vi "pp2_StimListPartition5.vi"(0 "Session List (Hidden variable)":u8[](array[numeric])=[0, 1, 2, 3, 4, 5, 6, 7, 8, 9, 10, 11, 12, 13, 14, 15, 100]) -> (7 "Session list display":string[][](table))   [LabVIEW 2013]
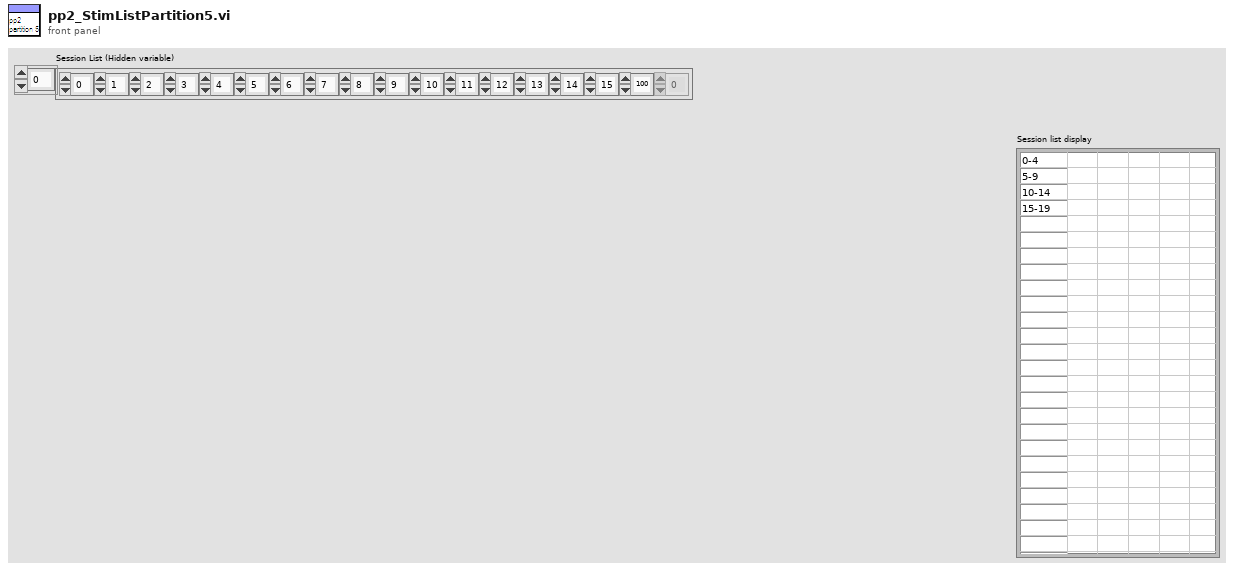
[diagram p1: front panel]
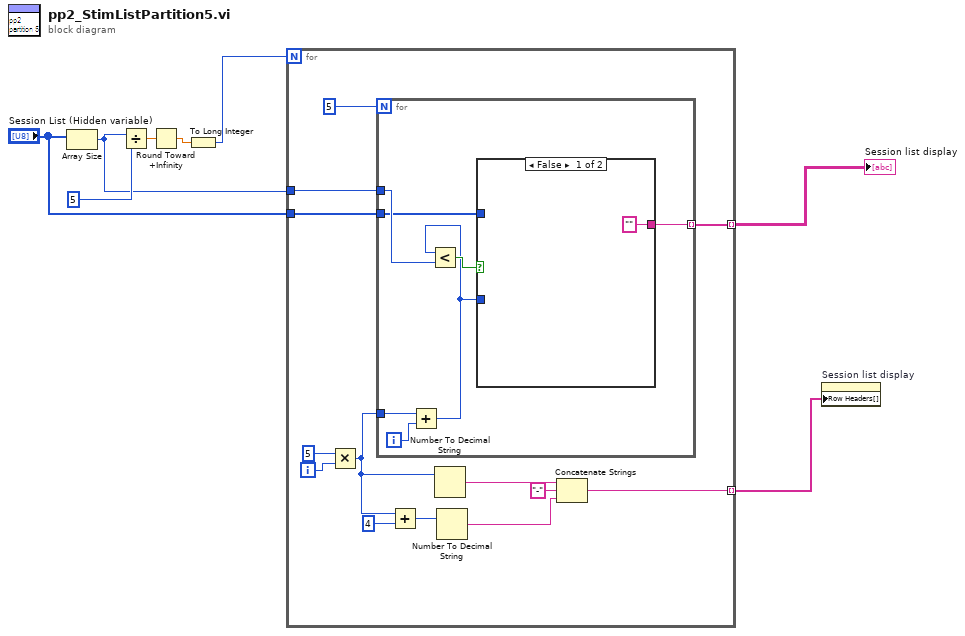
[diagram p0: block diagram]
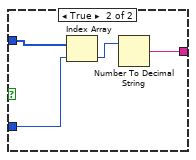
[diagram p2: hidden frame]
diagram:
  n1 = Array Size(array="Session List (Hidden variable)") -> (size(s)=w3:i32)
  n2 = Divide(x=w3, y=5) -> (x/y=w7:dbl)
  n3 = Round Toward +Infinity(x=w7) -> (ceil(x): smallest int >= x=w6:dbl)
  n4 = To Long Integer(number=w6) -> (32bit integer=w5:i32)
  n5 = for {
    N: w5 -> [_]
    tunnel: "Session List (Hidden variable)" -> [w20]
    tunnel: w3 -> [w19]
    tunnel: [w16] -> w2 mode=indexing
    tunnel: [w9] -> w1 mode=indexing
    i -> [w18]
    n6 = Multiply(x=5, y=w18) -> (x*y=w14:i32)
    n7 = for {
      N: 5 -> [_]
      tunnel: w20 -> [w24]
      tunnel: w19 -> [w25]
      tunnel: w14 -> [w27]
      tunnel: [w22] -> w16 mode=indexing
      i -> [w28]
      n8 = Add(x=w27, y=w28) -> (x+y=w23:i32)
      n9 = Less?(x=w23, y=w25) -> (x < y?=w26:bool)
      n10 = case shown="False" w26 {
        tunnel: w24 -> [_ w33]
        tunnel: w23 -> [_ w32]
        tunnel: ["" w30] -> w22
        frame False {
        }
        frame True {
          n11 = Index Array(array=w33, index=w32) -> (element=w31:u8)
          n12 = Number To Decimal String(number=w31) -> (decimal integer string=w30:string)  [unwired: 1 in]
        }
      }
    }
    n13 = Add(x=w14, y=4) -> (x+y=w15:i32)
    n14 = Number To Decimal String(number=w14) -> (decimal integer string=w12:string)  [unwired: 1 in]
    n15 = Number To Decimal String(number=w15) -> (decimal integer string=w10:string)  [unwired: 1 in]
    n16 = Concatenate Strings(w12, "-" ("string"), w10) -> (w9:string)
  }
  "Session list display" <- w2
  n17 = property on="Session list display" class="Tbl (strict)"("Row Headers[]"=w1) -> ()  [unwired: 2 in, 2 out]
